vi "HTS_CONFIG.vi"(5 "Loader Settings":T1={"Sample Flow Rate (uL/s)"=1.0, "Sample Volume (uL)"=8.0, "Mixing Volume (uL)"=30, "Mixing Speed (uL/s)"=50, "Mix#"=3, "Wash Volume (uL)"=200, "INJECTION_MODE"=enum."HT"} {"Sample Volume (uL)" min=2.0 max=200.0 step=0.5; "Mixing Volume (uL)" min=5 max=100 step=5; "Mixing Speed (uL/s)" min=25 max=250 step=5; "Sample Flow Rate (uL/s)" min=0.5 max=3.0 step=0.5 format="%_2f"; "Mix#" min=0 max=5 step=1; "Wash Volume (uL)" min=200 max=800 step=20}, 6 "error IO":errorcluster, 9 "VISA resource IN":refnum<visa-resource-name>="HTS") -> (0 "Error OUT":errorcluster, 3 "VISA resource OUT":refnum<visa-resource-name>="HTS")   [LabVIEW 2009]
uses:
  HTS_LOADER_SETTINGS.ctl
  HTS_INJECTION_MODE.ctl
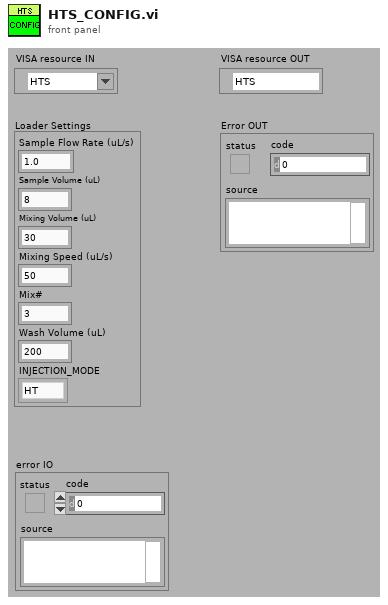
[diagram p1: front panel]
types:
  T1 = typedef "HTS_LOADER_SETTINGS.ctl" = cluster{"Sample Flow Rate (uL/s)":dbl, "Sample Volume (uL)":dbl, "Mixing Volume (uL)":i32, "Mixing Speed (uL/s)":i32, "Mix#":i32, "Wash Volume (uL)":i32, "INJECTION_MODE":T2}
  T2 = typedef "HTS_INJECTION_MODE.ctl" = enum16{"STD", "HT"}
  T3 = typedef "HTS_PMC_COMMAND_LIST.ctl" = string[][]
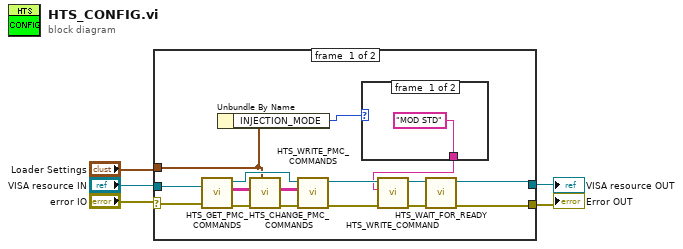
[diagram p0: block diagram]
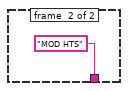
[diagram p2: hidden frame]
diagram:
  n1 = case shown="No Error" "error IO" {
    selector: "error IO" -> [w15 w24]
    tunnel: [w11 w25] -> w5
    tunnel: [w12 w24] -> w4
    tunnel: "VISA resource IN" -> [w16 w25]
    tunnel: "Loader Settings" -> [w8 _]
    frame #0 {
      n2 = call "HTS_GET_PMC_COMMANDS.vi"("Error IN"=w15, "VISA resource IN"=w16) -> ("Error OUT"=w18:errorcluster, "HTS_PMC_COMMANDS"=w20:T3, "VISA resource OUT"=w17:refnum<visa-resource-name>)  [unwired: 7 out]
      n3 = Unbundle By Name(w8) -> ("INJECTION_MODE"=w7:T2)
      n4 = call "HTS_CHANGE_PMC_COMMANDS.vi"("Loader Settings"=w8, "Error IN"=w18, "HTS_PMC_COMMAND_LIST"=w20) -> ("Error OUT"=w19:errorcluster, "NEW_PMC_COMMANDS"=w21:string[][])  [unwired: 7 out]
      n5 = call "HTS_WRITE_PMC_COMMANDS.vi"("Error IN"=w19, "HTS_PMC_COMMANDS"=w21, "VISA resource IN"=w17) -> ("Error OUT"=w13:errorcluster, "VISA resource OUT"=w9:refnum<visa-resource-name>)  [unwired: 7 out]
      n6 = case shown="\"STD\", Default" w7 {
        tunnel: ["MOD STD" "MOD HTS"] -> w6
        frame #0 {
        }
        frame #1 {
        }
      }
      n7 = call "HTS_WRITE_COMMAND.vi"("Error IN"=w13, "Command"=w6, "VISA resource IN"=w9) -> ("Error OUT"=w14:errorcluster, "VISA resource OUT"=w10:refnum<visa-resource-name>)  [unwired: 7 out]
      n8 = call "HTS_WAIT_FOR_READY.vi"("Error IN"=w14, "VISA resource IN"=w10) -> ("Error OUT"=w12:errorcluster, "VISA resource OUT"=w11:refnum<visa-resource-name>)  [unwired: 1 in, 7 out]
    }
    frame #1 {
    }
  }
  "VISA resource OUT" <- w5
  "Error OUT" <- w4
